vi "initialize_data_log.vi"(7 "Overwrite?":bool, 8 "error in (no error)":errorcluster, 9 "Initialization Data":variant, 10 "Path":path, 11 "scan_hdf5_log in":refnum<class "scan_hdf5_log.lvclass">) -> (0 "error out":errorcluster, 3 "scan_hdf5_log out":refnum<class "scan_hdf5_log.lvclass">)   [LabVIEW 2015, in "scan_hdf5_log.lvclass"]
uses:
  scan_hdf5_log.lvclass
  initialization_data.ctl
  scan_hdf5_log.lvclass/scan_hdf5_log.ctl
  <vilib>/UPVI/lvhdf5/dataset.llb/LVH5D Operation.ctl
  <vilib>/UPVI/lvhdf5/property.llb/LVH5PClassId.ctl
  <vilib>/UPVI/lvhdf5/file.llb/LVH5F Operation.ctl
  <vilib>/Utility/miscctls.llb/LVRectTypeDef.ctl
  <vilib>/UPVI/lvhdf5/group.llb/H5G_obj_t.ctl
  <vilib>/UPVI/lvhdf5/utility.llb/Select HDF5 Dialog.vi
  <vilib>/UPVI/lvhdf5/utility.llb/Select HDF5 Dialog (Object Only).vi
  <vilib>/UPVI/lvhdf5/dataset.llb/Simple H5Dwrite (Variant).vi
  <vilib>/UPVI/lvhdf5/datatype.llb/LVH5Tcreate_dataset_type (Variant).vi
  <vilib>/UPVI/lvhdf5/dataset.llb/Simple H5Dwrite.xnode
  <vilib>/UPVI/lvhdf5/library.llb/HDF5 Ref.ctl
  <vilib>/UPVI/lvhdf5/datatype.llb/LVH5Tcreate_dataset_type.xnode
  Detector_Class/Picoquant/Hydraharp/hydraharp/hydraharp.lvclass
  <vilib>/UPVI/lvhdf5/file.llb/H5Fclose.vi
  <vilib>/UPVI/lvhdf5/identifier.llb/Not an HDF5 Refnum Constant.vi
  <vilib>/Utility/error.llb/Error Cluster From Error Code.vi
  <vilib>/UPVI/lvhdf5/dataset.llb/OpenCreateReplace Dataset by Element Type.vi
  <vilib>/UPVI/lvhdf5/dataspace.llb/H5Sselect_hyperslab.vi
  <vilib>/UPVI/lvhdf5/dataset.llb/H5Dwrite (Variant).vi
  <vilib>/UPVI/lvhdf5/dataset.llb/H5Dget_space.vi
  <vilib>/UPVI/lvhdf5/attribute.llb/private/LVH5AwriteWDTAttrs.vi
  <vilib>/UPVI/lvhdf5/dataspace.llb/H5Sclose.vi
  <vilib>/UPVI/lvhdf5/utility.llb/Select HDF5 Dialog (File and Object).vi
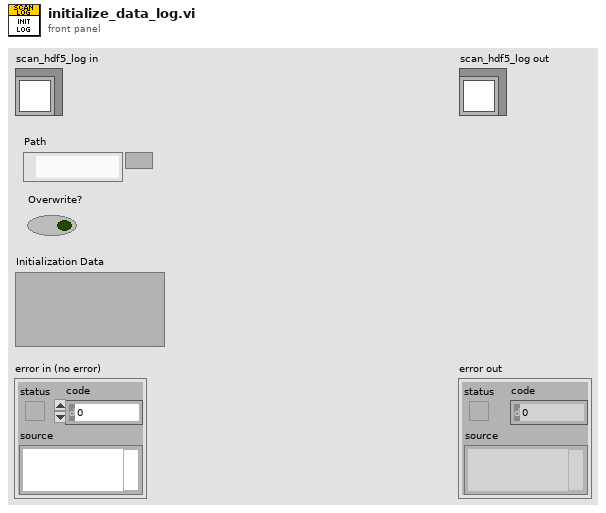
[diagram p1: front panel]
types:
  T1 = typedef "initialization_data.ctl" = cluster{"Positions (mm)":dbl[], "dims":u32[]}
  T2 = typedef "LVH5PClassId.ctl" = enum32{"H5P_ROOT", "H5P_OBJECT_CREATE", "H5P_FILE_CREATE", "H5P_FILE_ACCESS", "H5P_DATASET_CREATE", "H5P_DATASET_ACCESS", "H5P_DATASET_XFER", "H5P_FILE_MOUNT", "H5P_GROUP_CREATE", "H5P_GROUP_ACCESS", "H5P_DATATYPE_CREATE", "H5P_DATATYPE_ACCESS", "H5P_STRING_CREATE", "H5P_ATTRIBUTE_CREATE", "H5P_OBJECT_COPY", "H5P_LINK_CREATE", "H5P_LINK_ACCESS"}
  T3 = typedef "LVH5D Operation.ctl" = enum16{"open", "replace", "create", "open or create", "create or replace", "create or replace with confirmation"}
  T4 = typedef "LVH5F Operation.ctl" = enum16{"open", "open or create", "create or replace", "create or replace (with confirmation)", "create", "open (read only)"}
  T5 = typedef "LVRectTypeDef.ctl" = cluster{"Left":i16, "Top":i16, "Right":i16, "Bottom":i16}
  T6 = cluster{"Behavior":enum32{"Invalid", "Default", "Floating", "Floating/Auto-Hide", "Modal"}, "Position":T5, "Center":bool, "Title":string}
  T7 = typedef "H5G_obj_t.ctl" = i32
  T8 = cluster{"Object Types (any)":T7[], "Object Pattern":string}
  T9 = typedef "HDF5 Ref.ctl" = refnum<k1>
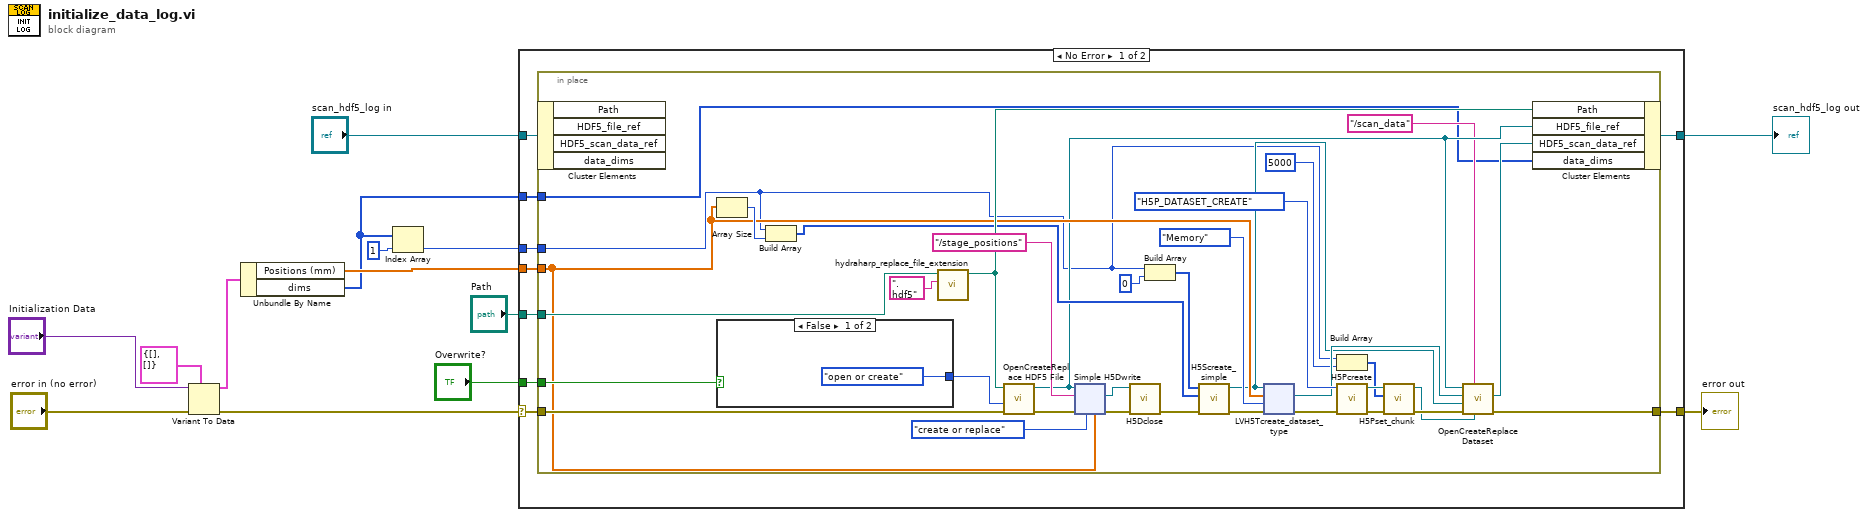
[diagram p0: block diagram]
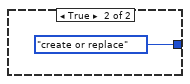
[diagram p2: hidden frame]
diagram:
  n1 = Variant To Data(error in="error in (no error)", type=T1 {"Positions (mm)"=[], "dims"=[]} ("output cluster"), Variant="Initialization Data") -> (data=w5:T1, error out=w12:errorcluster)
  n2 = Unbundle By Name(w5) -> ("Positions (mm)"=w4:dbl[], "dims"=w1:u32[])
  n3 = Index Array(array=w1, index=1) -> (element=w2:u32)
  n4 = case shown="No Error" w12 {
    selector: w12 -> [w20 w288]
    tunnel: w4 -> [w23 _]
    tunnel: "scan_hdf5_log in" -> [w22 w287]
    tunnel: "Overwrite?" -> [w21 _]
    tunnel: [w19 w287] -> w9
    tunnel: "Path" -> [w18 _]
    tunnel: [w17 w288] -> w7
    tunnel: w2 -> [w16 _]
    tunnel: w1 -> [w15 _]
    frame No Error {
      n5 = in-place {
        in-place-border: w23 -> [w43]
        in-place-border: w21 -> [w55]
        in-place-border: w20 -> [w53]
        in-place-border: w18 -> [w50]
        in-place-border: [w31] -> w17
        in-place-border: w16 -> [w26]
        in-place-border: w15 -> [w24]
        n6 = in-place-cluster #1(w22) -> ()  [unwired: 4 out]
        n7 = Array Size(array=w43) -> (size(s)=w46:i32)
        n8 = case shown="False" w55 {
          tunnel: [LVH5F_Operation."open or create" ("function (open or create)") LVH5F_Operation."create or replace" ("function (open or create)")] -> w54
          frame False {
          }
          frame True {
          }
        }
        n9 = Build Array(w26, w46) -> (w45:u32[])
        n10 = call "hydraharp_replace_file_extension.vi"("new_extension"=".hdf5", "input_file"=w50) -> ("new_name"=w51:path)  [unwired: 9 in]
        n11 = call <vilib>:"OpenCreateReplace HDF5 File.vi"("error in (no error)"=w53, "function (open or create)"=w54, "path"=w51) -> ("error out"=w52:errorcluster, "HDF5 Ref out"=w35:T9)  [unwired: 5 in]
        n12 = xnode "Simple H5Dwrite"("Dataset Path"="/stage_positions", "error in (no error)"=w52, "operation (open or create)"=LVH5D_Operation."create or replace", "HDF5 Path or Ref"=w35, "Data"=w43) -> ("HDF5 Dataset Ref out"=w49:T9, "error out"=w48:errorcluster)  [unwired: 3 in, 1 out]
        n13 = call <vilib>:"H5Dclose.vi"("error in (no error)"=w48, "HDF5 Dataset Ref"=w49) -> ("error out"=w47:errorcluster)  [unwired: 7 in]
        n14 = Build Array(w26, u32 0 ("element")) -> (w29:u32[])
        n15 = call <vilib>:"H5Screate_simple.vi"("error in (no error)"=w47, "Maximum Dimensions (unlimited)"=w45, "Dimensions"=w29) -> ("error out"=w44:errorcluster, "HDF5 Ref out"=w33:T9)  [unwired: 5 in]
        n16 = xnode "LVH5Tcreate_dataset_type"("HDF5 Location Ref"=w33, "Type"=enum16{"File", "Memory"}."Memory", "error in (no error)"=w44, "Data"=w43) -> ("HDF5 Type Ref"=w34:T9, "error out"=w39:errorcluster)  [unwired: 2 in, 3 out]
        n17 = Build Array(w26, u32 5000 ("element")) -> (w27:u32[])
        n18 = call <vilib>:"H5Pcreate.vi"("error in (no error)"=w39, "Property List Class"=LVH5PClassId."H5P_DATASET_CREATE") -> ("error out"=w41:errorcluster, "HDF5 Property List Ref"=w37:T9)  [unwired: 6 in]
        n19 = call <vilib>:"H5Pset_chunk.vi"("error in (no error)"=w41, "Dimensions"=w27, "HDF5 Property Ref"=w37) -> ("error out"=w38:errorcluster, "HDF5 Ref out"=w36:T9)  [unwired: 5 in]
        n20 = call <vilib>:"OpenCreateReplace Dataset.vi"("HDF5 Property List Ref"=w36, "Dataset Path"="/scan_data", "error in (no error)"=w38, "HDF5 Dataspace Ref"=w33, "HDF5 Datatype Ref"=w34, "HDF5 Ref"=w35) -> ("error out"=w31:errorcluster, "HDF5 Dataset Ref"=w30:T9)  [unwired: 3 in, 1 out]
        n21 = in-place-cluster #1("Path"=w51, "HDF5_file_ref"=w35, "HDF5_scan_data_ref"=w30, "data_dims"=w24) -> (w19:refnum<class "scan_hdf5_log.lvclass">)
      }
    }
    frame Error {
    }
  }
  "error out" <- w7
  "scan_hdf5_log out" <- w9
